vi "Handle Events.vi"(8 "error in (no error)":errorcluster, 11 "VIEventHandler":refnum<class "VIEventHandler.lvclass">) -> ()   [LabVIEW 2015, in "ActorEvents.lvlib" / "VIEventHandler.lvclass"]
uses:
  VIEventHandler.lvclass
  IEventHandler/IEventHandler.lvclass/IEventHandler.ctl
  VIEventHandler.lvclass/VIEventHandler.ctl
  <vilib>/ActorFramework/Message Enqueuer/Message Enqueuer.lvclass/Message Enqueuer.ctl
  <vilib>/ActorFramework/Message Priority Queue/Priority Enqueue.vi
  IEventHandler/IEventHandler.lvclass
  IEventAggregator Messages/UserMenuSelectionMsg/UserMenuSelectionMsg.lvclass
  IEventAggregator Messages/PanelCloseMsg/PanelCloseMsg.lvclass
  <vilib>/ActorFramework/Message Enqueuer/Message Enqueuer.lvclass
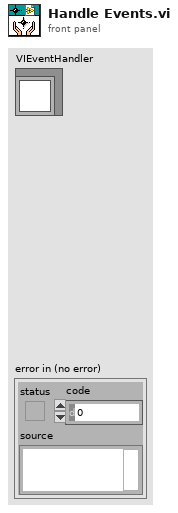
[diagram p1: front panel]
types:
  T1 = typedef "Actor Framework.lvlib/Message Enqueuer.lvclass/Message Priority.ctl" = enum16{"Low", "Normal", "High"}
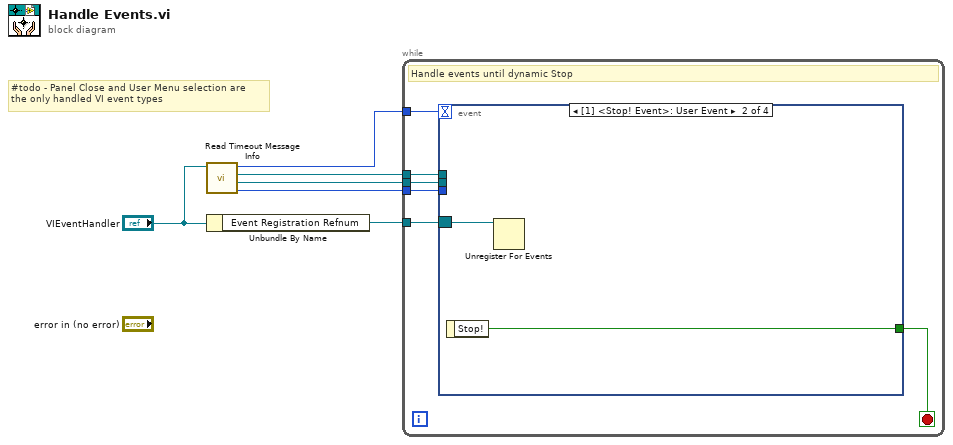
[diagram p0: block diagram]
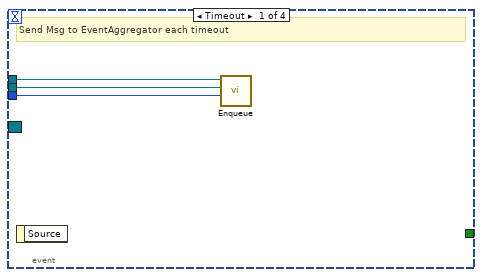
[diagram p2: hidden frame]
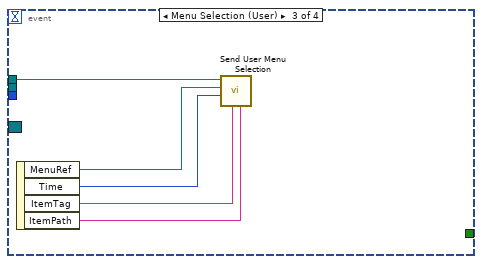
[diagram p3: hidden frame]
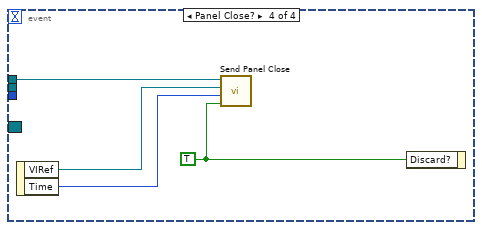
[diagram p4: hidden frame]
diagram:
  # "#todo - Panel Close and User Menu selection are\nthe only handled VI event types"
  n1 = call "Read Timeout Message Info.vi"("IEventHandler in"="VIEventHandler") -> ("Timeout Message Priority"=w2:T1, "Timeout Message"=w3:refnum<class "Message.lvclass">, "EventAggregator Enqueuer"=w4:refnum<class "Message Enqueuer.lvclass">, "Timeout [ms]"=w1:i32)  [unwired: 7 in]
  n2 = Unbundle By Name("VIEventHandler") -> ("Event Registration Refnum"=w6:refnum<event-registration>)
  n3 = while {
    tunnel: w6 -> [w12]
    tunnel: w4 -> [w10]
    tunnel: w3 -> [w9]
    tunnel: w2 -> [w8]
    tunnel: w1 -> [w7]
    stop <- w11 stop-if-true
    # "Handle events until dynamic Stop"
    n4 = event shown="[1] <Stop! Event>: User Event" {
      selector: w12 -> [_ w16 _ _]
      dyn-events: _ -> [_ _ _ _]
      timeout: w7 -> [_ _ _ _]
      tunnel: [_ w17 _ _] -> w11
      tunnel: w10 -> [w15 _ w22 w26]
      tunnel: w9 -> [w14 _ _ _]
      tunnel: w8 -> [w13 _ _ _]
      event Timeout {
        # "Send Msg to EventAggregator each timeout"
        n5 = event-data() -> ()  [unwired: 1 in, 1 out]
        n6 = call <vilib>:"Enqueue.vi"("Message Priority (Normal)"=w13, "Message"=w14, "Message Enqueuer in"=w15) -> ()  [unwired: 7 in, 2 out]
      }
      event User Event {
        n7 = event-data() -> ("Stop!"=w17:bool)  [unwired: 1 in]
        n8 = Unregister For Events(event registration refnum=w16) -> ()  [unwired: 1 in, 1 out]
      }
      event Menu Selection (User) {
        n9 = event-data() -> ("MenuRef"=w21:refnum<k9>, "Time"=w20:u32, "ItemTag"=w19:string, "ItemPath"=w18:string)  [unwired: 1 in]
        n10 = call "Send User Menu Selection.vi"("Item Path"=w18, "Item Tag"=w19, "Time"=w20, "MenuRef"=w21, "Message Enqueuer in"=w22) -> ()  [unwired: 6 in, 1 out]
      }
      event Panel Close? {
        w23 = TRUE ("Discarded?")
        n11 = event-data() -> ("VIRef"=w25:refnum<vi>, "Time"=w24:u32)  [unwired: 1 in]
        n12 = call "Send Panel Close.vi"("Discarded?"=w23, "Time"=w24, "VI Refnum"=w25, "Message Enqueuer in"=w26) -> ()  [unwired: 7 in, 1 out]
        n13 = event-data("Discard?"=w23) -> ()  [unwired: 1 in, 1 out]
      }
    }
  }
